vi "CRYResonance partial derivative.vi"(1 "x":dbl format="%.2f", 2 "Coefficients":dbl[](array[numeric]) format="%.2f") -> (0 "Partial Derivative":dbl[](array[numeric]) format="%.5f")   [LabVIEW 2013]
panel:
  # "Partial Derivative"
  # "This VI takes an input x along with a number of coefficients to use in the Target Func NonLin vi and does a numerical computation of the partial derivative of the function with repect to each coefficient at value x."
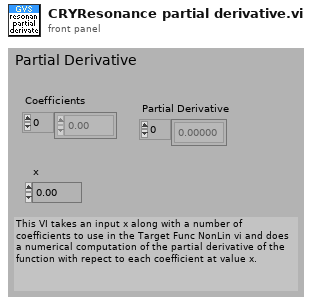
[diagram p1: front panel]
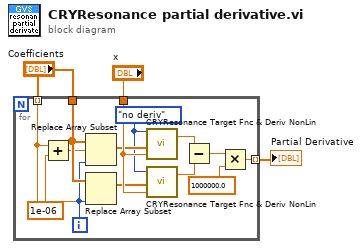
[diagram p0: block diagram]
diagram:
  n1 = for {
    tunnel: "x" -> [w10]
    tunnel: [w15] -> w2 mode=indexing
    tunnel: "Coefficients" -> [w9] mode=indexing
    tunnel: "Coefficients" -> [w13]
    i -> [w11]
    w4 = enum16{"no deriv", "deriv"}."no deriv"
    n2 = Add(x=w9, y=1e-06) -> (x+y=w12:dbl)
    n3 = Replace Array Subset(array=w13, new element=w12, index=w11) -> (w7:dbl[])
    n4 = Replace Array Subset(array=w13, new element=w9, index=w11) -> (w5:dbl[])
    n5 = call "CRYResonance Target Fnc & Deriv NonLin.vi"("X"=w10, "Coefficients"=w7, "Flag"=w4) -> ("Y"=w8:dbl)  [unwired: 1 out]
    n6 = call "CRYResonance Target Fnc & Deriv NonLin.vi"("X"=w10, "Coefficients"=w5, "Flag"=w4) -> ("Y"=w6:dbl)  [unwired: 1 out]
    n7 = Subtract(x=w8, y=w6) -> (x-y=w16:dbl)
    n8 = Multiply(x=w16, y=1000000.0) -> (x*y=w15:dbl)
  }
  "Partial Derivative" <- w2
